vi "QSM Queue Mgr SubVI 2.vi"(0 "QSTATES":cluster{"FN":T1, "Data":variant}[](array[cluster]), 2 "QRef":refnum<queue>, 11 "Error IN":errorcluster, 12 "FNs":enum16{"Back", "Front", "Replace"}(ring)) -> (15 "Error OUT":errorcluster)   [LabVIEW 2015]
uses:
  ctlSeqFNs_SubVI 2.ctl
  GLOBAL -MAIN.vi
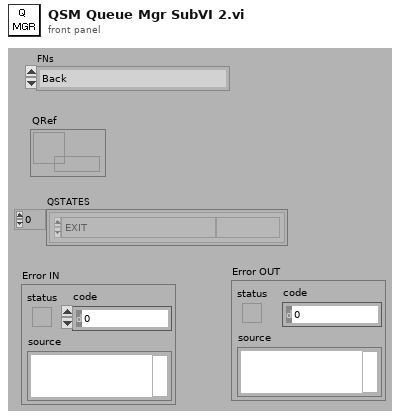
[diagram p1: front panel]
types:
  T1 = typedef "ctlSeqFNs_SubVI 2.ctl" = enum16{"INITIALIZE", "IDLE", "Convert deg F to deg C", "Send to Main", "Main Event Msg", "ERROR", "EXIT"}
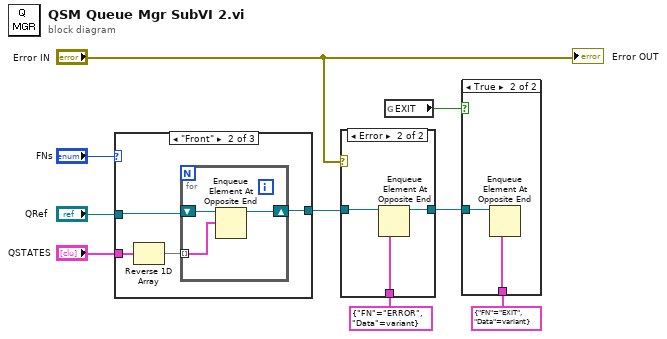
[diagram p0: block diagram]
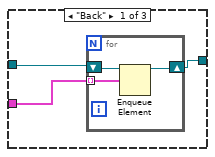
[diagram p4: hidden frame]
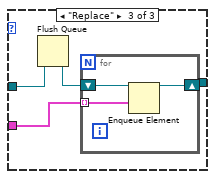
[diagram p5: hidden frame]
diagram:
  n1 = case shown="\"Front\"" "FNs" {
    tunnel: "QSTATES" -> [w10 w19 w24]
    tunnel: "QRef" -> [w12 w17 w26]
    tunnel: [w11 w16 w23] -> w6
    frame "Back" {
      n2 = for {
        shift-right: [w14] -> w11
        shift-left: w12 -> [w15]
        tunnel: w10 -> [w13] mode=indexing
        n3 = Enqueue Element(queue=w15, element=w13) -> (queue out=w14:refnum<queue>)  [unwired: 2 in, 2 out]
      }
    }
    frame "Front" {
      n4 = Reverse 1D Array(array=w19) -> (reversed array=w18:cluster{"FN":T1, "Data":variant}[])
      n5 = for {
        tunnel: w18 -> [w21] mode=indexing
        shift-right: [w20] -> w16
        shift-left: w17 -> [w22]
        n6 = Enqueue Element At Opposite End(queue=w22, element=w21) -> (queue out=w20:refnum<queue>)  [unwired: 2 in, 2 out]
      }
    }
    frame "Replace" {
      n7 = Flush Queue(queue=w26) -> (queue out=w25:refnum<queue>)  [unwired: 1 in, 2 out]
      n8 = for {
        tunnel: w24 -> [w28] mode=indexing
        shift-right: [w27] -> w23
        shift-left: w25 -> [w29]
        n9 = Enqueue Element(queue=w29, element=w28) -> (queue out=w27:refnum<queue>)  [unwired: 2 in, 2 out]
      }
    }
  }
  n10 = case shown="Error" "Error IN" {
    tunnel: w6 -> [w30 w33]
    tunnel: [w30 w32] -> w5
    tunnel: cluster{"FN":T1, "Data":variant} {"FN"=enum."ERROR", "Data"=variant} ("element") -> [_ w31]
    frame No Error {
    }
    frame Error {
      n11 = Enqueue Element At Opposite End(queue=w33, element=w31) -> (queue out=w32:refnum<queue>)  [unwired: 2 in, 2 out]
    }
  }
  n12 = global read "GLOBAL -MAIN.vi" "EXIT"() -> (w2:bool)
  n13 = case shown="True" w2 {
    tunnel: w5 -> [_ w35]
    tunnel: cluster{"FN":T1, "Data":variant} {"FN"=enum."EXIT", "Data"=variant} ("element") -> [_ w34]
    frame False {
    }
    frame True {
      n14 = Enqueue Element At Opposite End(queue=w35, element=w34) -> ()  [unwired: 2 in, 3 out]
    }
  }
  "Error OUT" <- "Error IN"
